vi "update.vi"(8 "error in (no error)":errorcluster, 10 "Model in":refnum<class "Model.lvclass">, 11 "PerformOpenLoopScanState in":refnum<class "PerformClosedLoopScanState.lvclass">) -> (0 "error out":errorcluster, 2 "Model out":refnum<class "Model.lvclass">, 3 "PerformOpenLoopScanState out":refnum<class "PerformClosedLoopScanState.lvclass">)   [LabVIEW 2015, in "PerformClosedLoopScanState.lvclass"]
uses:
  PerformClosedLoopScanState.lvclass
  Model/Model/Model.lvclass
  Typedefs/StateSelector.ctl
  Typedefs/FAMTTypedefs.lvlib
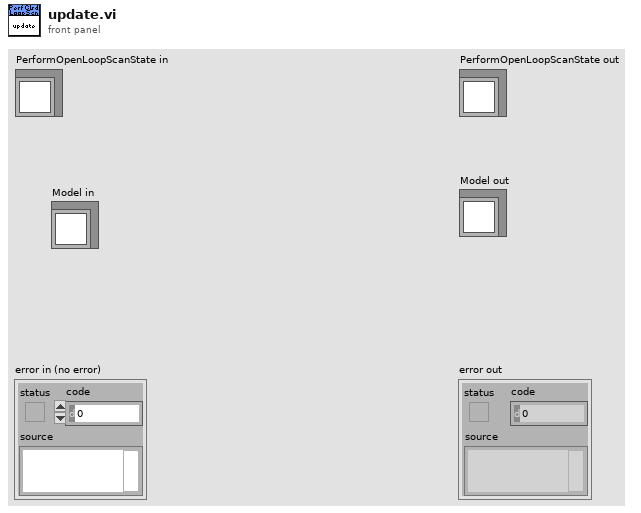
[diagram p1: front panel]
types:
  T1 = typedef "FAMTTypedefs.lvlib/StateSelector.ctl" = enum16{"OfflineState", "FaultState", "StandbyState", "DisabledState", "EnabledState", "WaitForUserInputState", "PerformOpenLoopScanState", "PerformClosedLoopScanState"}
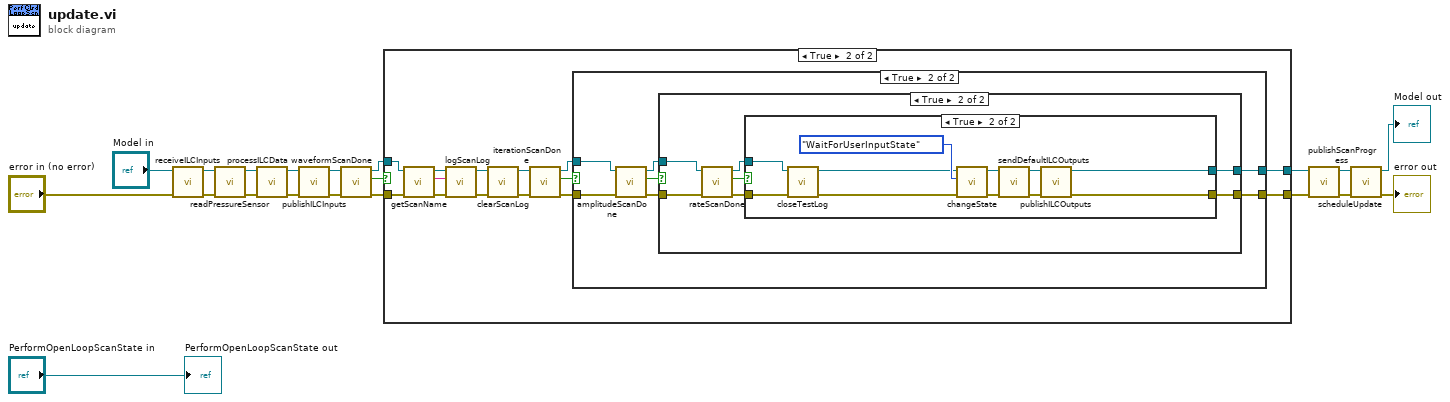
[diagram p0: block diagram]
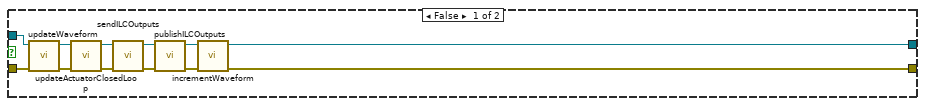
[diagram p2: hidden frame]
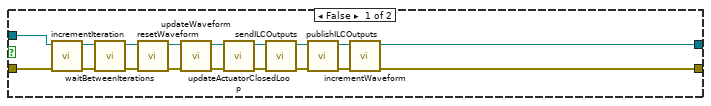
[diagram p3: hidden frame]
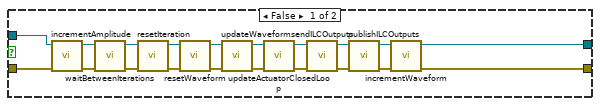
[diagram p4: hidden frame]
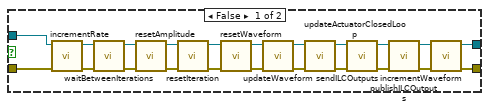
[diagram p5: hidden frame]
diagram:
  n1 = call "receiveILCInputs.vi"("error in (no error)"="error in (no error)", "Model in"="Model in") -> ("error out"=w9:errorcluster, "Model out"=w12:refnum<class "Model.lvclass">)  [unwired: 8 in]
  n2 = call "readPressureSensor.vi"("error in (no error)"=w9, "Model in"=w12) -> ("error out"=w8:errorcluster, "Model out"=w11:refnum<class "Model.lvclass">)  [unwired: 8 in]
  n3 = call "processILCData.vi"("error in (no error)"=w8, "Model in"=w11) -> ("error out"=w7:errorcluster, "Model out"=w20:refnum<class "Model.lvclass">)  [unwired: 8 in]
  n4 = call "publishILCInputs.vi"("error in (no error)"=w7, "Model in"=w20) -> ("error out"=w6:errorcluster, "Model out"=w14:refnum<class "Model.lvclass">)  [unwired: 8 in]
  n5 = call "waveformScanDone.vi"("error in (no error)"=w6, "Model in"=w14) -> ("error out"=w5:errorcluster, "Done?"=w16:bool, "Model out"=w15:refnum<class "Model.lvclass">)  [unwired: 7 in]
  n6 = case shown="True" w16 {
    tunnel: w15 -> [w27 w40]
    tunnel: [w21 w33] -> w4
    tunnel: [w29 w46] -> w13
    tunnel: w5 -> [w26 w38]
    frame False {
      n7 = call "updateWaveform.vi"("error in (no error)"=w26, "Model in"=w27) -> ("error out"=w25:errorcluster, "Model out"=w28:refnum<class "Model.lvclass">)  [unwired: 8 in]
      n8 = call "updateActuatorClosedLoop.vi"("error in (no error)"=w25, "Model in"=w28) -> ("error out"=w24:errorcluster, "Model out"=w32:refnum<class "Model.lvclass">)  [unwired: 8 in]
      n9 = call "sendILCOutputs.vi"("error in (no error)"=w24, "Model in"=w32) -> ("error out"=w23:errorcluster, "Model out"=w31:refnum<class "Model.lvclass">)  [unwired: 8 in]
      n10 = call "publishILCOutputs.vi"("error in (no error)"=w23, "Model in"=w31) -> ("error out"=w22:errorcluster, "Model out"=w30:refnum<class "Model.lvclass">)  [unwired: 8 in]
      n11 = call "incrementWaveform.vi"("error in (no error)"=w22, "Model in"=w30) -> ("error out"=w21:errorcluster, "Model out"=w29:refnum<class "Model.lvclass">)  [unwired: 8 in]
    }
    frame True {
      n12 = call "getScanName.vi"("error in (no error)"=w38, "Model in"=w40) -> ("error out"=w37:errorcluster, "Scan Name"=w39:string, "Model out"=w41:refnum<class "Model.lvclass">)  [unwired: 7 in]
      n13 = call "logScanLog.vi"("error in (no error)"=w37, "File Name"=w39, "Model in"=w41) -> ("error out"=w36:errorcluster, "Model out"=w43:refnum<class "Model.lvclass">)  [unwired: 7 in]
      n14 = call "clearScanLog.vi"("error in (no error)"=w36, "Model in"=w43) -> ("error out"=w35:errorcluster, "Model out"=w42:refnum<class "Model.lvclass">)  [unwired: 8 in]
      n15 = call "iterationScanDone.vi"("error in (no error)"=w35, "Model in"=w42) -> ("error out"=w34:errorcluster, "Done?"=w45:bool, "Model out"=w44:refnum<class "Model.lvclass">)  [unwired: 7 in]
      n16 = case shown="True" w45 {
        tunnel: w44 -> [w58 w69]
        tunnel: [w47 w65] -> w33
        tunnel: [w59 w68] -> w46
        tunnel: w34 -> [w55 w67]
        frame False {
          n17 = call "incrementIteration.vi"("error in (no error)"=w55, "Model in"=w58) -> ("error out"=w54:errorcluster, "Model out"=w57:refnum<class "Model.lvclass">)  [unwired: 8 in]
          n18 = call "waitBetweenIterations.vi"("error in (no error)"=w54, "Model in"=w57) -> ("error out"=w53:errorcluster, "Model out"=w56:refnum<class "Model.lvclass">)  [unwired: 8 in]
          n19 = call "resetWaveform.vi"("error in (no error)"=w53, "Model in"=w56) -> ("error out"=w52:errorcluster, "Model out"=w60:refnum<class "Model.lvclass">)  [unwired: 8 in]
          n20 = call "updateWaveform.vi"("error in (no error)"=w52, "Model in"=w60) -> ("error out"=w51:errorcluster, "Model out"=w61:refnum<class "Model.lvclass">)  [unwired: 8 in]
          n21 = call "updateActuatorClosedLoop.vi"("error in (no error)"=w51, "Model in"=w61) -> ("error out"=w50:errorcluster, "Model out"=w64:refnum<class "Model.lvclass">)  [unwired: 8 in]
          n22 = call "sendILCOutputs.vi"("error in (no error)"=w50, "Model in"=w64) -> ("error out"=w49:errorcluster, "Model out"=w63:refnum<class "Model.lvclass">)  [unwired: 8 in]
          n23 = call "publishILCOutputs.vi"("error in (no error)"=w49, "Model in"=w63) -> ("error out"=w48:errorcluster, "Model out"=w62:refnum<class "Model.lvclass">)  [unwired: 8 in]
          n24 = call "incrementWaveform.vi"("error in (no error)"=w48, "Model in"=w62) -> ("error out"=w47:errorcluster, "Model out"=w59:refnum<class "Model.lvclass">)  [unwired: 8 in]
        }
        frame True {
          n25 = call "amplitudeScanDone.vi"("error in (no error)"=w67, "Model in"=w69) -> ("error out"=w66:errorcluster, "Done?"=w71:bool, "Model out"=w70:refnum<class "Model.lvclass">)  [unwired: 7 in]
          n26 = case shown="True" w71 {
            tunnel: w70 -> [w91 w97]
            tunnel: [w72 w92] -> w65
            tunnel: [w87 w95] -> w68
            tunnel: w66 -> [w81 w94]
            frame False {
              n27 = call "incrementAmplitude.vi"("error in (no error)"=w81, "Model in"=w91) -> ("error out"=w80:errorcluster, "Model out"=w83:refnum<class "Model.lvclass">)  [unwired: 8 in]
              n28 = call "waitBetweenIterations.vi"("error in (no error)"=w80, "Model in"=w83) -> ("error out"=w79:errorcluster, "Model out"=w82:refnum<class "Model.lvclass">)  [unwired: 8 in]
              n29 = call "resetIteration.vi"("error in (no error)"=w79, "Model in"=w82) -> ("error out"=w78:errorcluster, "Model out"=w84:refnum<class "Model.lvclass">)  [unwired: 8 in]
              n30 = call "resetWaveform.vi"("error in (no error)"=w78, "Model in"=w84) -> ("error out"=w77:errorcluster, "Model out"=w86:refnum<class "Model.lvclass">)  [unwired: 8 in]
              n31 = call "updateWaveform.vi"("error in (no error)"=w77, "Model in"=w86) -> ("error out"=w76:errorcluster, "Model out"=w85:refnum<class "Model.lvclass">)  [unwired: 8 in]
              n32 = call "updateActuatorClosedLoop.vi"("error in (no error)"=w76, "Model in"=w85) -> ("error out"=w75:errorcluster, "Model out"=w90:refnum<class "Model.lvclass">)  [unwired: 8 in]
              n33 = call "sendILCOutputs.vi"("error in (no error)"=w75, "Model in"=w90) -> ("error out"=w74:errorcluster, "Model out"=w89:refnum<class "Model.lvclass">)  [unwired: 8 in]
              n34 = call "publishILCOutputs.vi"("error in (no error)"=w74, "Model in"=w89) -> ("error out"=w73:errorcluster, "Model out"=w88:refnum<class "Model.lvclass">)  [unwired: 8 in]
              n35 = call "incrementWaveform.vi"("error in (no error)"=w73, "Model in"=w88) -> ("error out"=w72:errorcluster, "Model out"=w87:refnum<class "Model.lvclass">)  [unwired: 8 in]
            }
            frame True {
              n36 = call "rateScanDone.vi"("error in (no error)"=w94, "Model in"=w97) -> ("error out"=w93:errorcluster, "Done?"=w98:bool, "Model out"=w96:refnum<class "Model.lvclass">)  [unwired: 7 in]
              n37 = case shown="True" w98 {
                tunnel: w96 -> [w117 w127]
                tunnel: [w99 w121] -> w92
                tunnel: [w116 w128] -> w95
                tunnel: w93 -> [w109 w125]
                frame False {
                  n38 = call "incrementRate.vi"("error in (no error)"=w109, "Model in"=w117) -> ("error out"=w108:errorcluster, "Model out"=w111:refnum<class "Model.lvclass">)  [unwired: 8 in]
                  n39 = call "waitBetweenIterations.vi"("error in (no error)"=w108, "Model in"=w111) -> ("error out"=w107:errorcluster, "Model out"=w110:refnum<class "Model.lvclass">)  [unwired: 8 in]
                  n40 = call "resetAmplitude.vi"("error in (no error)"=w107, "Model in"=w110) -> ("error out"=w106:errorcluster, "Model out"=w113:refnum<class "Model.lvclass">)  [unwired: 8 in]
                  n41 = call "resetIteration.vi"("error in (no error)"=w106, "Model in"=w113) -> ("error out"=w105:errorcluster, "Model out"=w112:refnum<class "Model.lvclass">)  [unwired: 8 in]
                  n42 = call "resetWaveform.vi"("error in (no error)"=w105, "Model in"=w112) -> ("error out"=w104:errorcluster, "Model out"=w115:refnum<class "Model.lvclass">)  [unwired: 8 in]
                  n43 = call "updateWaveform.vi"("error in (no error)"=w104, "Model in"=w115) -> ("error out"=w103:errorcluster, "Model out"=w114:refnum<class "Model.lvclass">)  [unwired: 8 in]
                  n44 = call "updateActuatorClosedLoop.vi"("error in (no error)"=w103, "Model in"=w114) -> ("error out"=w102:errorcluster, "Model out"=w120:refnum<class "Model.lvclass">)  [unwired: 8 in]
                  n45 = call "sendILCOutputs.vi"("error in (no error)"=w102, "Model in"=w120) -> ("error out"=w101:errorcluster, "Model out"=w119:refnum<class "Model.lvclass">)  [unwired: 8 in]
                  n46 = call "publishILCOutputs.vi"("error in (no error)"=w101, "Model in"=w119) -> ("error out"=w100:errorcluster, "Model out"=w118:refnum<class "Model.lvclass">)  [unwired: 8 in]
                  n47 = call "incrementWaveform.vi"("error in (no error)"=w100, "Model in"=w118) -> ("error out"=w99:errorcluster, "Model out"=w116:refnum<class "Model.lvclass">)  [unwired: 8 in]
                }
                frame True {
                  n48 = call "closeTestLog.vi"("error in (no error)"=w125, "Model in"=w127) -> ("error out"=w124:errorcluster, "Model out"=w126:refnum<class "Model.lvclass">)  [unwired: 8 in]
                  n49 = call "changeState.vi"("error in (no error)"=w124, "State:"=StateSelector."WaitForUserInputState", "Model in"=w126) -> ("error out"=w123:errorcluster, "Model out"=w130:refnum<class "Model.lvclass">)  [unwired: 7 in]
                  n50 = call "sendDefaultILCOutputs.vi"("error in (no error)"=w123, "Model in"=w130) -> ("error out"=w122:errorcluster, "Model out"=w129:refnum<class "Model.lvclass">)  [unwired: 8 in]
                  n51 = call "publishILCOutputs.vi"("error in (no error)"=w122, "Model in"=w129) -> ("error out"=w121:errorcluster, "Model out"=w128:refnum<class "Model.lvclass">)  [unwired: 8 in]
                }
              }
            }
          }
        }
      }
    }
  }
  n52 = call "publishScanProgress.vi"("error in (no error)"=w4, "Model in"=w13) -> ("error out"=w3:errorcluster, "Model out"=w17:refnum<class "Model.lvclass">)  [unwired: 8 in]
  n53 = call "scheduleUpdate.vi"("error in (no error)"=w3, "Model in"=w17) -> ("error out"=→"error out":errorcluster, "Model out"=→"Model out":refnum<class "Model.lvclass">)  [unwired: 8 in]
  "PerformOpenLoopScanState out" <- "PerformOpenLoopScanState in"
